vi "Send REGISTER.vi"(8 "REGISTER request data":T1, 9 "Message Loop Shift Register Data":T2, 10 "error in (no error)":errorcluster, 11 "WAMP Client in":refnum<class "WAMP Client.lvclass">) -> (1 "Message Loop Shift Register Data":T2, 2 "error out":errorcluster, 3 "WAMP Client out":refnum<class "WAMP Client.lvclass">)   [LabVIEW 2020, in "wamplv.lvlib" / "WAMP Client.lvclass"]
uses:
  WAMP Client.lvclass
  TypeDef/Message Loop Shift Reg Data.ctl
  TypeDef/REGISTER Request Data.ctl
  TypeDef/Success or error.ctl
  API/TypeDefs/Combined error.ctl
  API/TypeDefs/WAMP error.ctl
  API/TypeDefs/INVOCATION payload.ctl
  TypeDef/Publish Requests Map.ctl
  TypeDef/PUBLISH Request Data.ctl
  TypeDef/PUBLISH result.ctl
  TypeDef/Endpoint Data.ctl
  TypeDef/CALL Request Map.ctl
  TypeDef/CALL Request Data.ctl
  API/TypeDefs/RESULT payload.ctl
  TypeDef/SUBSCRIBE Requests Map.ctl
  TypeDef/SUBSCRIBE Request Data.ctl
  TypeDef/Subscribe Result.ctl
  TypeDef/EVENT payload.ctl
  TypeDef/Subscriptions Map.ctl
  TypeDef/Subscription Details.ctl
  TypeDef/Unsubscribe Requests Map.ctl
  TypeDef/UNSUBSCRIBE Request Data.ctl
  TypeDef/UNSUBSCRIBE Result.ctl
  TypeDef/Unregister requests map.ctl
  TypeDef/Unregister request.ctl
  TypeDef/WAMP Message Codes.ctl
  WAMP Client.lvclass/WAMP Client.ctl
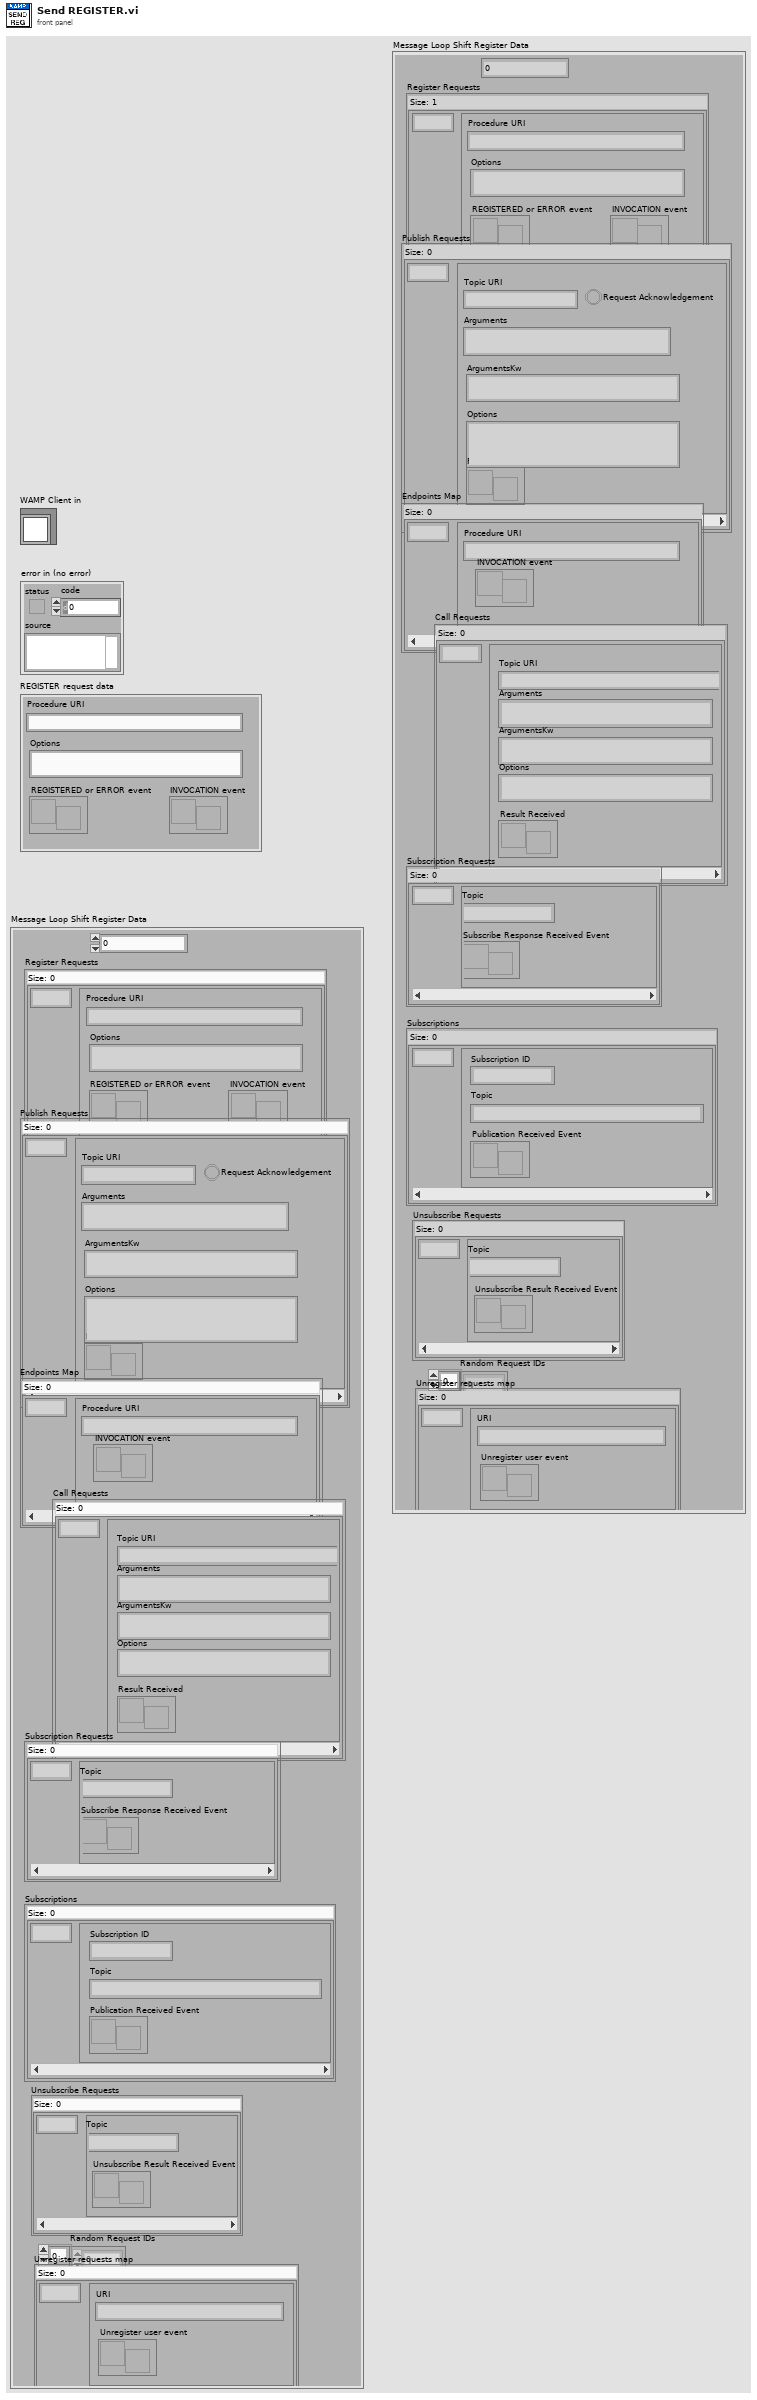
[diagram p1: front panel]
types:
  T1 = typedef "wamplv.lvlib/WAMP Client.lvclass/REGISTER Request Data.ctl" = cluster{"Procedure URI":string, "Options":string, "REGISTERED or ERROR event":refnum<user-event>, "INVOCATION event":refnum<user-event>}
  T2 = typedef "wamplv.lvlib/WAMP Client.lvclass/Message Loop Shift Reg Data.ctl" = cluster{"Last Request ID":u64, "Register Requests":map{u64, T1}, "Publish Requests":T3, "Endpoints Map":map{u64, T5}, "Call Requests":T6, "Subscription Requests":T8, "Subscriptions":T10, "Unsubscribe Requests":T12, "Random Request IDs":u64[], "Unregister requests map":T14}
  T3 = typedef "wamplv.lvlib/WAMP Client.lvclass/Publish Requests Map.ctl" = map{u64, T4}
  T4 = typedef "wamplv.lvlib/WAMP Client.lvclass/PUBLISH Request Data.ctl" = cluster{"Topic URI":string, "Arguments":string, "ArgumentsKw":string, "Publish Result Event":refnum<user-event>, "Request Acknowledgement":bool, "Options":string}
  T5 = typedef "wamplv.lvlib/WAMP Client.lvclass/Endpoint Data.ctl" = cluster{"Procedure URI":string, "INVOCATION event":refnum<user-event>}
  T6 = typedef "wamplv.lvlib/WAMP Client.lvclass/CALL Request Map.ctl" = map{u64, T7}
  T7 = typedef "wamplv.lvlib/WAMP Client.lvclass/CALL Request Data.ctl" = cluster{"Topic URI":string, "Arguments":string, "ArgumentsKw":string, "Result Received":refnum<user-event>, "Options":string}
  T8 = typedef "wamplv.lvlib/WAMP Client.lvclass/SUBSCRIBE Requests Map.ctl" = map{u64, T9}
  T9 = typedef "wamplv.lvlib/WAMP Client.lvclass/SUBSCRIBE Request Data.ctl" = cluster{"Topic":string, "Subscribe Response Received Event":refnum<user-event>}
  T10 = typedef "wamplv.lvlib/WAMP Client.lvclass/Subscriptions Map.ctl" = map{u64, T11}
  T11 = typedef "wamplv.lvlib/WAMP Client.lvclass/Subscription Details.ctl" = cluster{"Subscription ID":u64, "Topic":string, "Publication Received Event":refnum<user-event>}
  T12 = typedef "wamplv.lvlib/WAMP Client.lvclass/Unsubscribe Requests Map.ctl" = map{u64, T13}
  T13 = typedef "wamplv.lvlib/WAMP Client.lvclass/UNSUBSCRIBE Request Data.ctl" = cluster{"Topic":string, "Unsubscribe Result Received Event":refnum<user-event>}
  T14 = typedef "wamplv.lvlib/WAMP Client.lvclass/Unregister requests map.ctl" = map{u64, T15}
  T15 = typedef "wamplv.lvlib/WAMP Client.lvclass/Unregister request.ctl" = cluster{"URI":string, "Unregister user event":refnum<user-event>}
  T16 = typedef "wamplv.lvlib/WAMP Client.lvclass/WAMP Message Codes.ctl" = u16
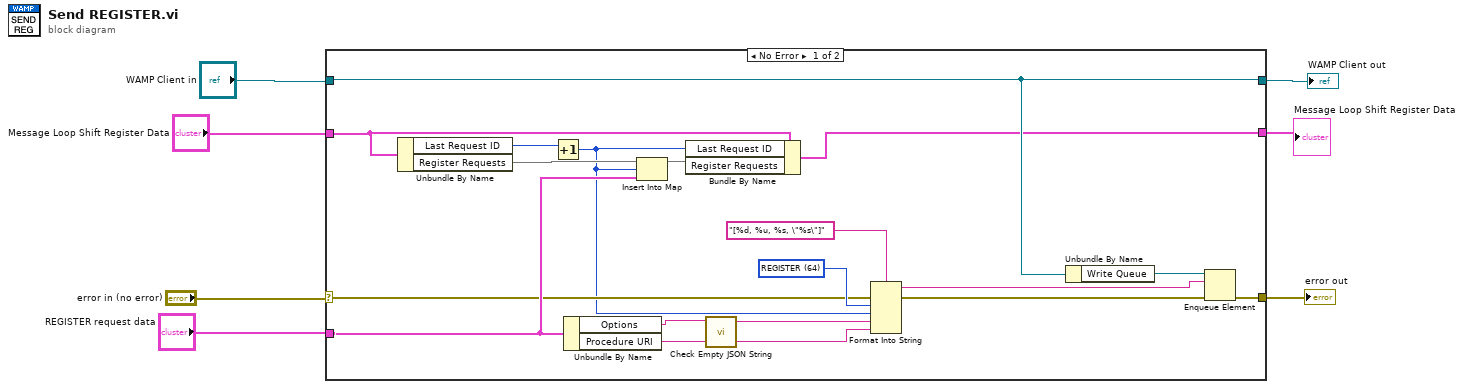
[diagram p0: block diagram]
diagram:
  n1 = case shown="No Error" "error in (no error)" {
    selector: "error in (no error)" -> [w12 w28]
    tunnel: [w20 w28] -> w6
    tunnel: [w21 w27] -> w4
    tunnel: "WAMP Client in" -> [w21 w27]
    tunnel: "REGISTER request data" -> [w16 _]
    tunnel: "Message Loop Shift Register Data" -> [w15 w26]
    tunnel: [w13 w26] -> w1
    frame No Error {
      w22 = T16 64 items=["HELLO"=1, "WELCOME"=2, "ABORT"=3, "GOODBYE"=6, "ERROR"=8, "PUBLISH"=16, "PUBLISHED"=17, "SUBSCRIBE"=32, "SUBSCRIBED"=33, "UNSUBSCRIBE"=34, "UNSUBSCRIBED"=35, "EVENT"=36, "CALL"=48, "RESULT"=59, "REGISTER"=64, "REGISTERED"=65, "UNREGISTER"=66, "UNREGISTERED"=67, "INVOCATION"=68, "YIELD"=70] ("Message Codes")
      n2 = Unbundle By Name(w15) -> ("Last Request ID"=w9:u64, "Register Requests"=w17:map{u64, T1})
      n3 = Increment(x=w9) -> (x+1=w8:u64)
      n4 = Unbundle By Name(w16) -> ("Options"=w11:string, "Procedure URI"=w18:string)
      n5 = Insert Into Map(map in=w17, key=w8, value=w16) -> (map out=w14:map{u64, T1})  [unwired: 2 out]
      n6 = Bundle By Name(cluster=w15, "Last Request ID"=w8, "Register Requests"=w14) -> (w13:T2)
      n7 = call "Check Empty JSON String.vi"("JSON"=w11) -> ("JSON"=w10:string)  [unwired: 10 in]
      n8 = Format Into String(format string="[%d, %u, %s, \"%s\"]" ("element"), error in=w12, w22, w8, w10, w18) -> (resulting string=w24:string, error out=w25:errorcluster)  [unwired: 1 in]
      n9 = Unbundle By Name(w21) -> ("Write Queue"=w19:refnum<queue>)
      n10 = Enqueue Element(queue=w19, element=w24, error in (no error)=w25) -> (error out=w20:errorcluster)  [unwired: 1 in, 2 out]
    }
    frame Error {
    }
  }
  "error out" <- w6
  "WAMP Client out" <- w4
  "Message Loop Shift Register Data" <- w1
